vi "Write Multiline.vi"(8 "error in (no error)":errorcluster, 10 "Multiline (T)":bool=TRUE, 11 "Serializer.JSON in":refnum<class "Serializer.JSON.lvclass">) -> (0 "error out":errorcluster, 3 "Serializer.JSON out":refnum<class "Serializer.JSON.lvclass">)   [LabVIEW 2019, in "OpenSerializer.JKI-JSON.lvlib" / "Serializer.JSON.lvclass"]
uses:
  Serializer.JSON.lvclass
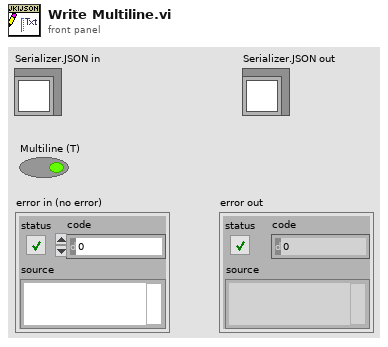
[diagram p1: front panel]
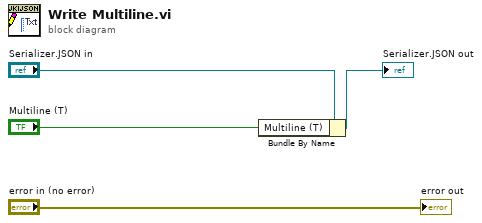
[diagram p0: block diagram]
diagram:
  n1 = Bundle By Name(cluster="Serializer.JSON in", "Multiline (T)"="Multiline (T)") -> (→"Serializer.JSON out":refnum<class "Serializer.JSON.lvclass">)
  "error out" <- "error in (no error)"
